vi "Handle.vi"(7 "Event jettl in":refnum<class "Event jettl.lvclass">, 11 "Nominal State in":refnum<class "Nominal State.lvclass">) -> (2 "Destroy?":bool, 5 "Event jettl out":refnum<class "Event jettl.lvclass">)   [LabVIEW 2021, in "jettl.lvlib" / "Base Event jettl.lvlib" / "Nominal State.lvclass"]
uses:
  Nominal State.lvclass
  Event jettl/Event jettl.lvclass
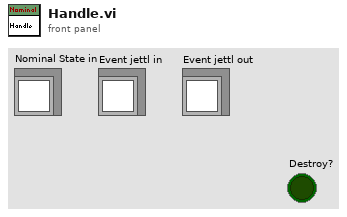
[diagram p1: front panel]
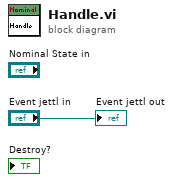
[diagram p0: block diagram]
diagram:
  "Event jettl out" <- "Event jettl in"
